vi "intro.vi"() -> ()   [LabVIEW 2012]
panel:
  in  "stop":bool
  in  "Acquire":bool
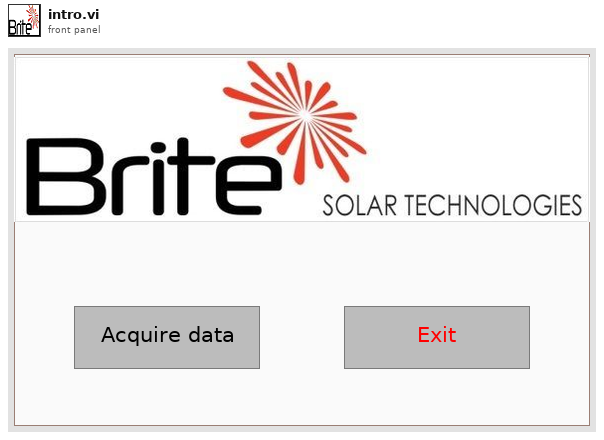
[diagram p1: front panel]
types:
  T1 = enum32{"Invalid", "Standard", "Closed", "Hidden", "Minimized", "Maximized"}
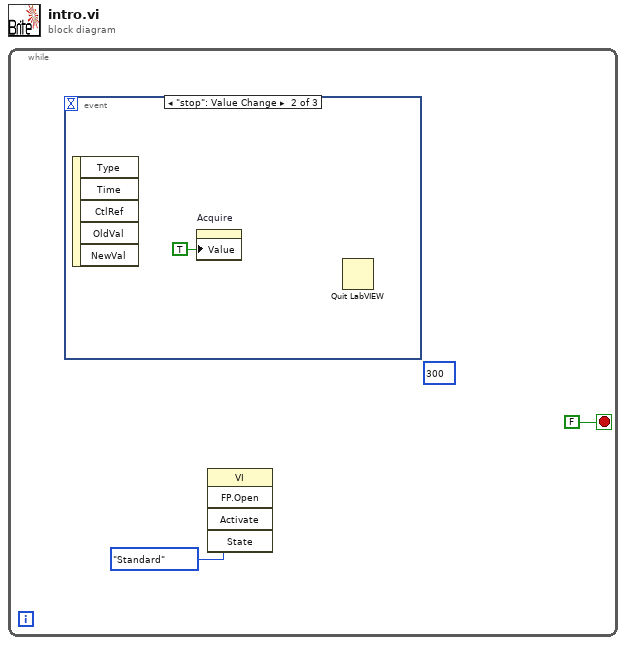
[diagram p0: block diagram]
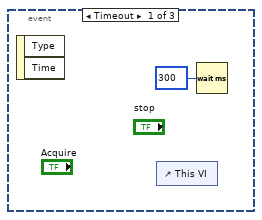
[diagram p2: hidden frame]
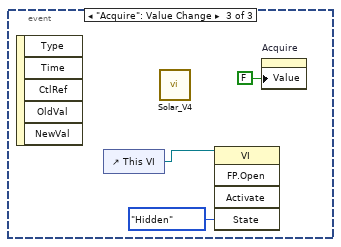
[diagram p3: hidden frame]
diagram:
  n1 = while {
    stop <- FALSE stop-if-true
    (unwired) u32 300 ("milliseconds to wait")
    n2 = event shown="[1] \"stop\": Value Change" {
      selector: _ -> [_ _ _]
      dyn-events: _ -> [_ _ _]
      timeout: _ -> [_ _ _]
      event Timeout {
        n3 = event-data() -> ()  [unwired: 1 in, 2 out]
        n4 = control-ref of="This VI"() -> ()  [unwired: 1 out]
        n5 = Wait (ms)(milliseconds to wait=u32 300) -> ()  [unwired: 1 out]
      }
      event "stop": Value Change {
        n6 = event-data() -> ()  [unwired: 1 in, 5 out]
        n7 = property on="Acquire" class="Bool (strict)"("Value"=TRUE ("Acquire")) -> ()  [unwired: 2 in, 2 out]
        n8 = Quit LabVIEW() -> ()  [unwired: 1 in]
      }
      event "Acquire": Value Change {
        n9 = event-data() -> ()  [unwired: 1 in, 5 out]
        n10 = control-ref of="This VI"() -> (w6:refnum<vi>)
        n11 = call "Solar_V4.vi"() -> ()  [unwired: 12 in]
        n12 = invoke class="VI" method="FP.Open"(reference=w6, "State"=T1."Hidden") -> ()  [unwired: 3 in, 5 out]
        n13 = property on="Acquire" class="Bool (strict)"("Value"=FALSE ("Acquire")) -> ()  [unwired: 2 in, 2 out]
      }
    }
    n14 = invoke class="VI" method="FP.Open"("State"=T1."Standard") -> ()  [unwired: 4 in, 5 out]
  }
